vi "Buffer (Data array Load) v1.00.vi"(0 "Read#":u8(slide)=1 min=1 step=1 scale=1.0..100.0) -> (2 "X-Data out":dbl[](array[numeric]) format="%.2f", 3 "Y-Data out":dbl[](array[numeric]) format="%.2f", 4 "WL unit 2":i32, 5 "Continue? 2":bool)   [LabVIEW 2021]
doc: "Write (FIFO) or retrieve (LIFO) data from the buffer.\n\nWhen write to the buffer, set the desired \"Buffer Size\" and run the VI several iterations. Notice that initially, the buffer grows to reach \"Buffer Size\" and then the input data flows from the last buffer element through to the zero element on each iteration (First In, First Out).\n\nWhen read from the buffer, set the Read# to the nth previous input data, i.e. counting reversely, with the most recent input counted as the 1st readout. If the input is out of current buffer size, an error is returned. (Last In, First Out)"
panel:
  in  "Boolean":bool=TRUE
  in  "Speed":u16(slide)=100 min=50 max=5000 step=50 scale=10.0..5000.0
  in  "Movie":bool
  out "File Contents":string
  in  "WL unit":i32(ring)=1 items=["Wavelength", "nm", "eV", "meV", "cm-1"]
  in  "Continue?":bool
  in  "Cancel":bool
  out "File Path":path
  out "?":T1(graph)
  # "Latest"
  # "Erliest"
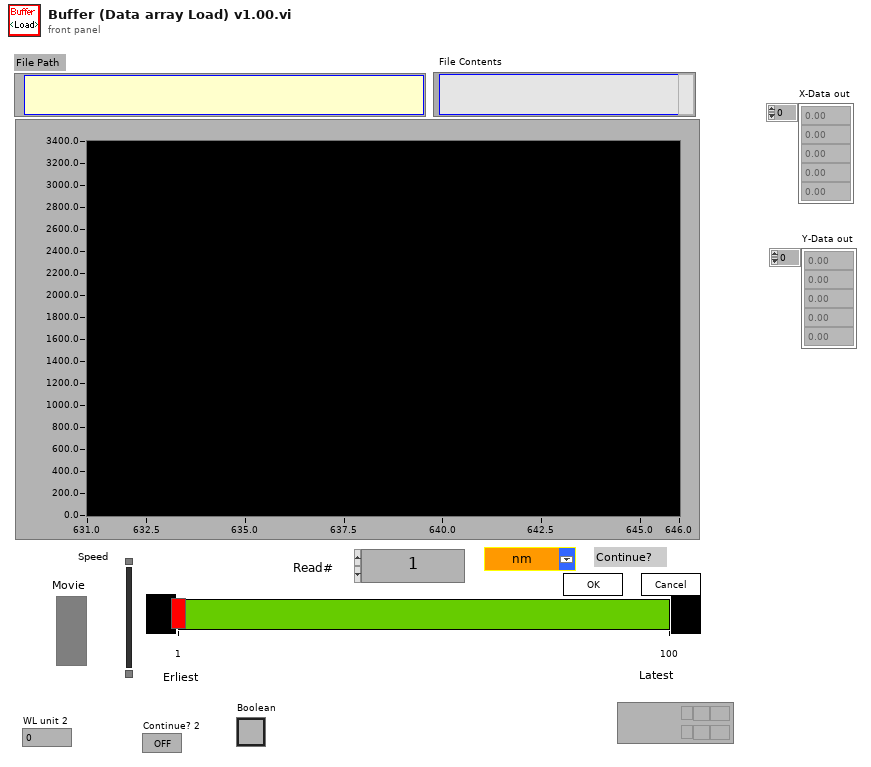
[diagram p1: front panel]
types:
  T1 = cluster{"Ramp Pattern":dbl[], "Sinc Pattern":dbl[]}
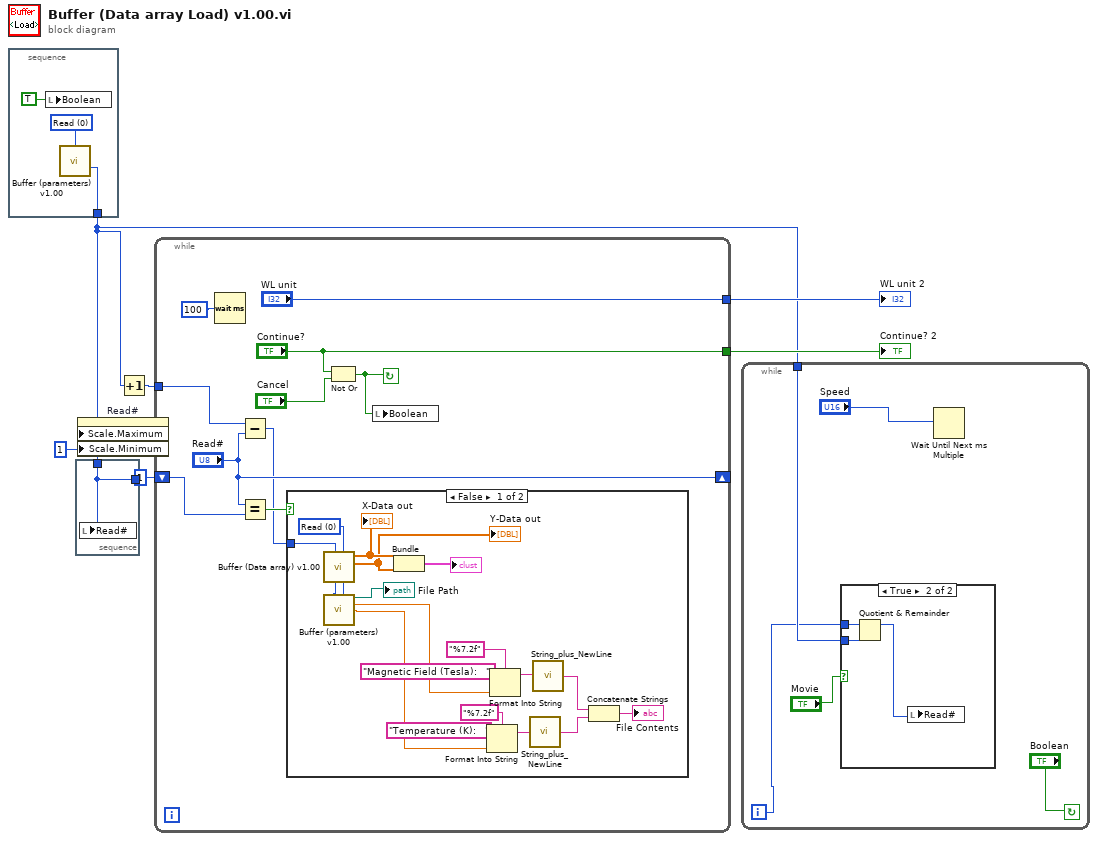
[diagram p0: block diagram]
diagram:
  n1 = stacked-sequence {
    tunnel: [w8] -> w2
    frame #0 {
      w9 = u16 0 items=["Read", "Write", "Initialize"] ("Read(0) or Write(1)")
      n2 = local write "Boolean"(TRUE ("Boolean")) -> ()
      n3 = call "Buffer (parameters) v1.00.vi"("Action"=w9) -> ("Current Buffer Size"=w8:i32)  [unwired: 10 in, 4 out]
    }
  }
  n4 = stacked-sequence {
    tunnel: w2 -> [w10]
    tunnel: [w10] -> _
    frame #0 {
      n5 = local write "Read#"(w10) -> ()
    }
  }
  n6 = property on="Read#" class="Slide (strict)"("Scale.Maximum"=w2, "Scale.Minimum"=u32 1 ("milliseconds to wait")) -> ()  [unwired: 2 in, 2 out]
  n7 = Increment(x=w2) -> (x+1=w3:i32)
  n8 = while {
    tunnel: w3 -> [w14]
    shift-left: u8 1 ("Read#") -> [w16]
    shift-right: ["Read#"] -> _
    tunnel: ["Continue?"] -> w5
    tunnel: ["WL unit"] -> w6
    stop <- w11 continue-if-true
    n9 = Wait (ms)(milliseconds to wait=u32 100) -> ()  [unwired: 1 out]
    n10 = Subtract(x=w14, y="Read#") -> (x-y=w12:i32)
    n11 = Equal?(x="Read#", y=w16) -> (x = y?=w15:bool)
    n12 = case shown="False" w15 {
      tunnel: w12 -> [w35 _]
      frame False {
        w36 = u16 0 items=["Read", "Write", "Initialize"] ("Read(0) or Write(1)")
        n13 = call "Buffer (Data array) v1.00.vi"("Action"=w36, "Read#"=w35) -> ("Y-Data out"=w21:dbl[], "X-Data out"=w22:dbl[])  [unwired: 6 in, 2 out]
        "X-Data out" <- w22
        "Y-Data out" <- w21
        n14 = call "Buffer (parameters) v1.00.vi"("Read#"=w35, "Action"=w36) -> ("FilePath out"=→"File Path":path, "Field Out"=w24:dbl, "Temperature Out"=w23:dbl)  [unwired: 9 in, 2 out]
        n15 = Bundle("X-Data out"=w22, "Y-Data out"=w21) -> (→"?":cluster{"X-Data out":dbl[], "Y-Data out":dbl[]})  [unwired: 1 in]
        n16 = Format Into String(format string="%7.2f", initial string="Temperature (K):   ", w23) -> (resulting string=w30:string)  [unwired: 1 in, 1 out]
        n17 = Format Into String(format string="%7.2f", initial string="Magnetic Field (Tesla):   ", w24) -> (resulting string=w32:string)  [unwired: 1 in, 1 out]
        n18 = call "String_plus_NewLine.vi"("Input String"=w30) -> ("Input String +[\\n]"=w26:string)
        n19 = call "String_plus_NewLine.vi"("Input String"=w32) -> ("Input String +[\\n]"=w27:string)
        n20 = Concatenate Strings(w27, w26) -> (→"File Contents":string)
      }
      frame True {
      }
    }
    n21 = Not Or(1:"Cancel", 2:"Continue?") -> (0:w11:bool)
    n22 = local write "Boolean"(w11) -> ()
  }
  "WL unit 2" <- w6
  "Continue? 2" <- w5
  n23 = while {
    tunnel: w2 -> [w42]
    i -> [w39]
    stop <- "Boolean" continue-if-true
    n24 = case shown="True" "Movie" {
      tunnel: w42 -> [_ w45]
      tunnel: w39 -> [_ w43]
      frame False {
      }
      frame True {
        n25 = Quotient & Remainder(x=w43, y=w45) -> (x-y*floor(x/y)=w44:i32)  [unwired: 1 out]
        n26 = local write "Read#"(w44) -> ()
      }
    }
    n27 = Wait Until Next ms Multiple(millisecond multiple="Speed") -> ()  [unwired: 1 out]
  }
